vi "setStrain.vi"(6 "Channel":i32, 8 "error in (no error)":errorcluster, 9 "Slew (V/s)":dbl, 10 "Strain (V)":dbl, 11 "Instrument.Strain in":refnum<class "Instrument.Strain.lvclass">) -> (0 "error out":errorcluster, 3 "Instrument.Strain out":refnum<class "Instrument.Strain.lvclass">)   [LabVIEW 2019, in "Instrument.Strain.lvclass"]
uses:
  Instrument.Strain.lvclass
  Typedefs/setStrain--cluster.ctl
  Typedefs/Strain.Commands--Enum.ctl
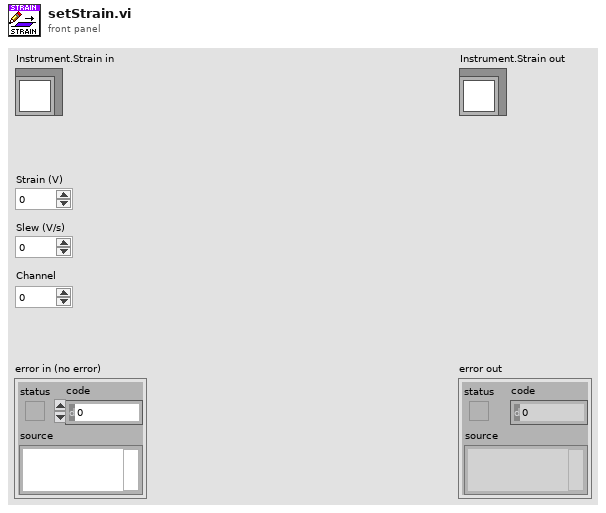
[diagram p1: front panel]
types:
  T1 = typedef "Instrument.Strain.lvclass/Strain.Commands--Enum.ctl" = enum16{"getStrain", "setStrain"}
  T2 = typedef "Instrument.Strain.lvclass/setStrain--cluster.ctl" = cluster{"strain":dbl, "slew":dbl, "channel":i32}
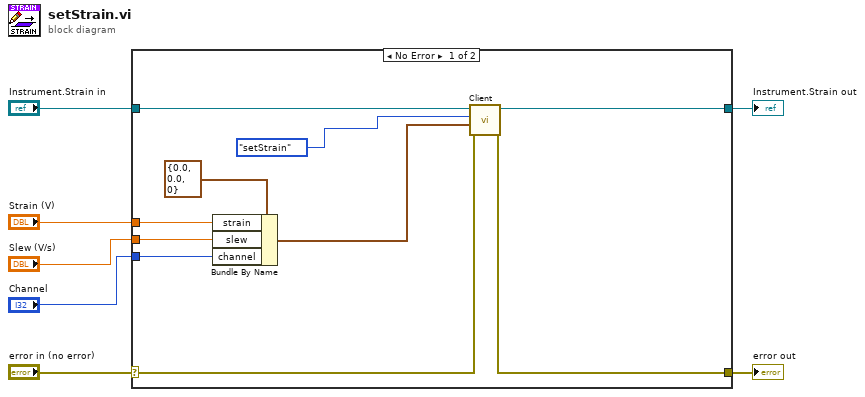
[diagram p0: block diagram]
diagram:
  n1 = case shown="No Error" "error in (no error)" {
    selector: "error in (no error)" -> [w9 w19]
    tunnel: [w16 w19] -> w6
    tunnel: [w17 w18] -> w4
    tunnel: "Instrument.Strain in" -> [w10 w18]
    tunnel: "Strain (V)" -> [w14 _]
    tunnel: "Slew (V/s)" -> [w13 _]
    tunnel: "Channel" -> [w12 _]
    frame No Error {
      n2 = Bundle By Name(cluster=T2 {"strain"=0.0, "slew"=0.0, "channel"=0} ("setStrain"), "strain"=w14, "slew"=w13, "channel"=w12) -> (w11:T2)
      n3 = call-dynamic "Client.vi"("error in (no error)"=w9, "Data in"=w11, "Command in"=Strain.Commands--Enum."setStrain" ("Command"), "Instrument in"=w10) -> ("error out"=w16:errorcluster, "Instrument out"=w17:refnum<class "Instrument.Strain.lvclass">)  [unwired: 4 in, 2 out]
    }
    frame Error {
    }
  }
  "error out" <- w6
  "Instrument.Strain out" <- w4
